vi "meas01.vi"() -> ()   [LabVIEW 2015]
uses:
  <vilib>/DAQmx/write.llb/DAQmx Write (Analog Wfm 1Chan NSamp).vi
  <vilib>/DAQmx/create/channels.llb/DAQmx Create Channel (AO-Voltage-Basic).vi
  <vilib>/DAQmx/configure/timing.llb/DAQmx Timing (Sample Clock).vi
  <vilib>/DAQmx/miscellaneous.llb/DAQmx Fill In Error Info.vi
  <vilib>/DAQmx/create/channels.llb/DAQmx Create Channel (CO-Pulse Generation-Frequency).vi
  <vilib>/DAQmx/configure/timing.llb/DAQmx Timing (Implicit).vi
  <vilib>/Utility/file.llb/Write Delimited Spreadsheet (DBL).vi
  <vilib>/measure/NI_MABase.lvlib
panel:
  in  "Vertical Coupling (1: DC)":i32(ring)=1 items=["AC", "DC", "Ground"]
  out "Waveform Data":waveform(dbl)(graph)
  out "Log-Log Frequency and Gain":cluster{"Y":dbl[], "Y":dbl[]}[](graph)
  out "freq in":dbl
  out "Loop #":i32
  out "detected amplitude":dbl format="%.2p"
  out "detected frequency":dbl format="%.2p"
  in  "Trigger Level (0.0 V)":dbl
  in  "Trigger Mode (0: Auto)":i32(ring) items=["Auto", "Normal"]
  in  "VISA resource name":refnum<visa-resource-name>
  in  "# Points":dbl
  in  "Highest Freq":dbl
  in  "Lowest Freq":dbl
  in  "Frequency (Hz)":dbl
  in  "Stop Clock":bool
  in  "Run":bool
  in  "stop":bool
  in  "physical channels":tag
  out "Amplitude":dbl
  in  "Amplitude":dbl(knob) scale=0.0..5.0
  in  "signal type":T1(ring)
  # "Clock"
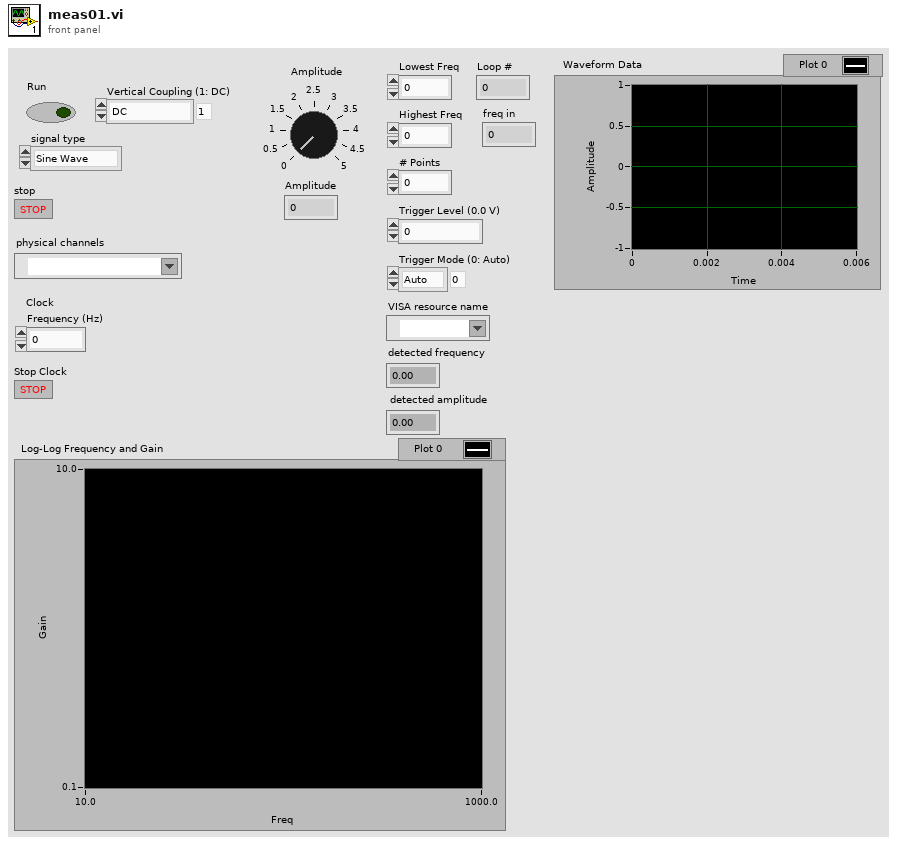
[diagram p1: front panel]
types:
  T1 = enum16{"Sine Wave", "Triangle Wave", "Square Wave", "Sawtooth Wave"}
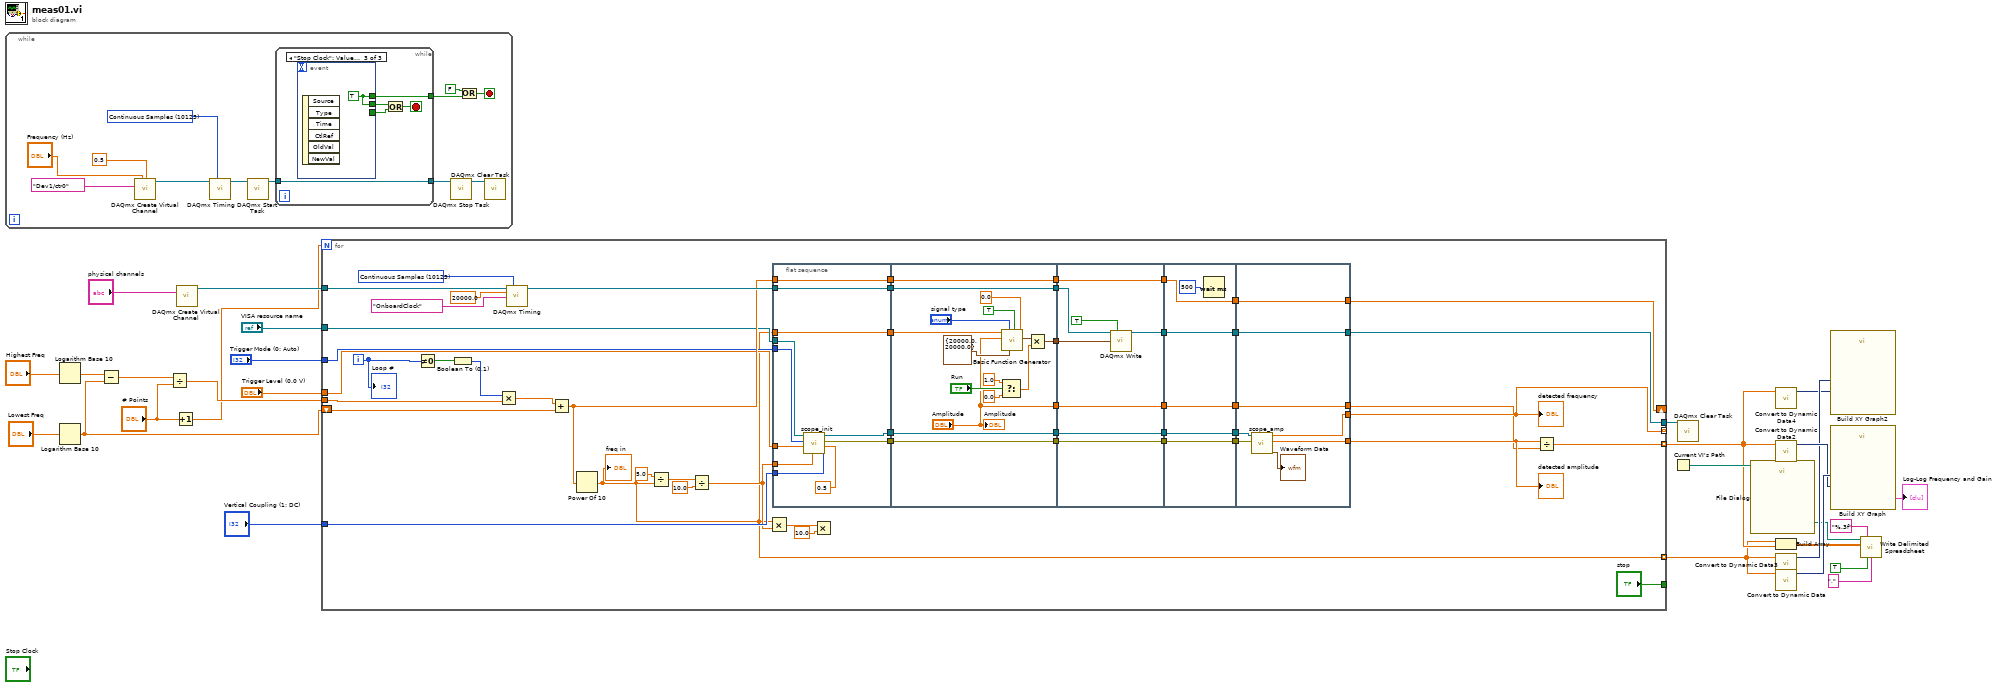
[diagram p0: block diagram]
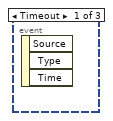
[diagram p2: hidden frame]
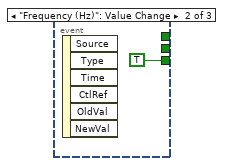
[diagram p3: hidden frame]
diagram:
  n1 = while {
    stop <- w32 stop-if-true
    w38 = 10123 items=["Finite Samples"=10178, "Continuous Samples"=10123, "Hardware Timed Single Point"=12522] ("sample mode")
    n2 = call-poly <vilib>:"DAQmx Create Virtual Channel.vi"("frequency"="Frequency (Hz)", "duty cycle"=0.5, "counter"=tag "Dev1/ctr0") -> ("task out"=w37:refnum<k21>)  [unwired: 11 in, 1 out]
    n3 = call-poly <vilib>:"DAQmx Timing.vi"("task/channels in"=w37, "sample mode"=w38) -> ("task out"=w36:refnum<k21>)  [unwired: 12 in, 1 out]
    n4 = call <vilib>:"DAQmx Start Task.vi"("task/channels in"=w36) -> ("task out"=w35:refnum<k21>)  [unwired: 13 in, 1 out]
    n5 = while {
      tunnel: w35 -> [w45]
      tunnel: [w45] -> w34
      tunnel: [w41] -> w31
      stop <- w42 stop-if-true
      n6 = event shown="[2] \"Stop Clock\": Value Change" {
        selector: _ -> [_ _ _]
        dyn-events: _ -> [_ _ _]
        timeout: _ -> [_ _ _]
        tunnel: [_ TRUE _] -> w43
        tunnel: [_ _ w47] -> w44
        tunnel: [_ _ w47] -> w41
        event Timeout {
          n7 = event-data() -> ()  [unwired: 1 in, 3 out]
        }
        event "Frequency (Hz)": Value Change {
          n8 = event-data() -> ()  [unwired: 1 in, 6 out]
        }
        event "Stop Clock": Value Change {
          w47 = TRUE
          n9 = event-data() -> ()  [unwired: 1 in, 6 out]
        }
      }
      n10 = Or(x=w44, y=w43) -> (x .or. y?=w42:bool)
    }
    n11 = call <vilib>:"DAQmx Stop Task.vi"("task/channels in"=w34) -> ("task out"=w33:refnum<k21>)  [unwired: 13 in, 1 out]
    n12 = Or(x=FALSE, y=w31) -> (x .or. y?=w32:bool)
    n13 = call <vilib>:"DAQmx Clear Task.vi"("task in"=w33) -> ()  [unwired: 14 in, 1 out]
  }
  n14 = Logarithm Base 10(1:"Highest Freq") -> (0:w20:dbl)
  n15 = Logarithm Base 10(1:"Lowest Freq") -> (0:w22:dbl)
  n16 = Subtract(x=w20, y=w22) -> (x-y=w24:dbl)
  n17 = Divide(x=w24, y="# Points") -> (x/y=w25:dbl)
  n18 = Increment(x="# Points") -> (x+1=w18:dbl)
  n19 = call-poly <vilib>:"DAQmx Create Virtual Channel.vi"("physical channels"="physical channels") -> ("task out"=w28:refnum<k21>)  [unwired: 13 in, 1 out]
  n20 = for {
    N: w18 -> [_]
    tunnel: w28 -> [w97]
    tunnel: [w74] -> w27
    tunnel: ["stop"] -> _
    tunnel: w25 -> [w92]
    tunnel: [w90] -> w2 mode=indexing
    tunnel: [w85] -> _ mode=indexing
    shift-right: [w66] -> _
    shift-left: w22 -> [w89]
    tunnel: "Trigger Level (0.0 V)" -> [w59]
    tunnel: "Trigger Mode (0: Auto)" -> [w61]
    tunnel: "VISA resource name" -> [w60]
    tunnel: "Vertical Coupling (1: DC)" -> [w58]
    tunnel: [w54] -> w1 mode=indexing
    i -> [w87]
    w94 = 10123 items=["Finite Samples"=10178, "Continuous Samples"=10123, "Hardware Timed Single Point"=12522] ("sample mode")
    n21 = Not Equal To 0?(x=w87) -> (x != 0?=w88:bool)
    n22 = Boolean To (0,1)(Boolean=w88) -> (0, 1=w86:i16)
    n23 = Multiply(x=w86, y=w92) -> (x*y=w91:dbl)
    n24 = call-poly <vilib>:"DAQmx Timing.vi"("task/channels in"=w97, "sample mode"=w94, "rate"=20000.0, "source"=tag "OnboardClock") -> ("task out"=w95:refnum<k21>)  [unwired: 10 in, 1 out]
    n25 = Add(x=w91, y=w89) -> (x+y=w67:dbl)
    n26 = Power Of 10(x=w67) -> (10^x=w54:dbl)
    "freq in" <- w54
    n27 = Divide(x=5.0, y=w54) -> (x/y=w78:dbl)
    n28 = Divide(x=w78, y=10.0) -> (x/y=w57:dbl)
    n29 = Multiply(x=w54, y=w57) -> (x*y=w56:dbl)
    n30 = flat-sequence {
      tunnel: w95 -> [w109]
      tunnel: [w109] -> w73
      tunnel: [w106] -> w72
      tunnel: [w105] -> w71
      tunnel: [w108] -> w68
      tunnel: w67 -> [w108]
      tunnel: [w107] -> w62
      tunnel: w54 -> [w107]
      tunnel: w61 -> [w101]
      tunnel: w60 -> [w104]
      tunnel: w59 -> [w102]
      tunnel: w57 -> [w103]
      tunnel: w58 -> [w99]
      tunnel: [w125] -> w53
      tunnel: [w124] -> w52
      tunnel: [w123] -> w51
      tunnel: w73 -> [w125]
      tunnel: w72 -> [w124]
      tunnel: w71 -> [w123]
      tunnel: [w122] -> w50
      tunnel: w68 -> [w122]
      tunnel: ["Amplitude"] -> w49
      tunnel: w62 -> [w121]
      tunnel: [w110] -> w48
      tunnel: [w132] -> w83
      tunnel: [w131] -> w81
      tunnel: [w130] -> w75
      tunnel: w53 -> [w133]
      tunnel: w52 -> [w132]
      tunnel: w51 -> [w131]
      tunnel: [w129] -> w69
      tunnel: w50 -> [w129]
      tunnel: [w128] -> w64
      tunnel: w49 -> [w128]
      tunnel: w48 -> [w126]
      tunnel: w83 -> [w139]
      tunnel: [w139] -> w82
      tunnel: w81 -> [w138]
      tunnel: [w138] -> w80
      tunnel: [w136] -> w76
      tunnel: w75 -> [w136]
      tunnel: [w135] -> w70
      tunnel: w69 -> [w135]
      tunnel: [w134] -> w65
      tunnel: w64 -> [w134]
      tunnel: w82 -> [w147]
      tunnel: w80 -> [w146]
      tunnel: [w145] -> w85
      tunnel: [w144] -> w84
      tunnel: [w143] -> w74
      tunnel: w76 -> [w143]
      tunnel: [w142] -> w66
      tunnel: w70 -> [w142]
      tunnel: [w141] -> w63
      tunnel: w65 -> [w141]
      frame #0 {
        n31 = call "scope_init.vi"("Vertical Coupling (1: DC)"=w99, "Vertical Range (10.0 V/div)"=0.5, "Timebase (0.0005 s)"=w103, "Trigger Level (0.0 V)"=w102, "Trigger Mode (0: Auto)"=w101, "VISA resource name"=w104) -> ("error out"=w105:errorcluster, "VISA resource name out"=w106:refnum<visa-resource-name>)  [unwired: 4 in]
      }
      frame #1 {
        n32 = Select(t=1.0, s="Run", f=0.0) -> (s? t:f=w116:dbl)
        n33 = call <vilib>:"Basic Function Generator.vi"("offset"=0.0, "reset signal"=TRUE, "sampling info"=cluster{"Fs":dbl, "#s":dbl} {"Fs"=20000.0, "#s"=20000.0}, "signal type"="signal type", "amplitude"="Amplitude", "frequency"=w121) -> ("signal out"=w120:waveform(dbl))  [unwired: 3 in, 2 out]
        n34 = Multiply(x=w120, y=w116) -> (x*y=w110:waveform(dbl))
        "Amplitude" <- "Amplitude"
      }
      frame #2 {
        n35 = call-poly <vilib>:"DAQmx Write.vi"("task/channels in"=w133, "auto start"=TRUE, "data"=w126) -> ("task out"=w130:refnum<k21>)  [unwired: 10 in, 2 out]
      }
      frame #3 {
        n36 = Wait (ms)(milliseconds to wait=u32 500) -> ()  [unwired: 1 out]
      }
      frame #4 {
        n37 = call "scope_amp.vi"("error in (no error)"=w146, "VISA resource name"=w147) -> ("Waveform Data"=→"Waveform Data":waveform(dbl), "detected amplitude"=w144:dbl, "detected frequency"=w145:dbl)  [unwired: 6 in, 1 out]
      }
    }
    n38 = Multiply(x=w56, y=10.0) -> ()  [unwired: 1 out]
    n39 = Divide(x=w84, y=w63) -> (x/y=w90:dbl)
    "detected frequency" <- w85
    "detected amplitude" <- w84
    "Loop #" <- w87
  }
  n40 = Current VI's Path() -> (path=w9:path)
  n41 = call <vilib>:"DAQmx Clear Task.vi"("task in"=w27) -> ()  [unwired: 14 in, 1 out]
  n42 = call "File Dialog"("start path"=w9) -> ("selected path"=w7:path)  [unwired: 11 in, 3 out]
  n43 = call "Convert to Dynamic Data4"("Array"=w2) -> ("Dynamic Data Type"=w13:dynamicdata)  [unwired: 3 in]
  n44 = call "Convert to Dynamic Data2"("Array"=w2) -> ("Dynamic Data Type"=w15:dynamicdata)  [unwired: 3 in]
  n45 = Build Array(w1, w2) -> (w4:dbl[][])
  n46 = call "Convert to Dynamic Data3"("Array"=w1) -> ("Dynamic Data Type"=w14:dynamicdata)  [unwired: 3 in]
  n47 = call "Convert to Dynamic Data"("Array"=w1) -> ("Dynamic Data Type"=w16:dynamicdata)  [unwired: 3 in]
  n48 = call "Build XY Graph2"("Y Input"=w13, "X Input"=w14) -> ()  [unwired: 8 in, 2 out]
  n49 = call "Build XY Graph"("Y Input"=w15, "X Input"=w16) -> ("XY Graph"=→"Log-Log Frequency and Gain":cluster{"X":dbl[], "Y":dbl[]}[])  [unwired: 8 in, 1 out]
  n50 = call-poly <vilib>:"Write Delimited Spreadsheet.vi"("file path (dialog if empty)"=w7, "format (%.3f)"="%.3f", "2D data"=w4, "transpose? (F)"=TRUE ("transpose? (no:F)"), "delimiter (\\t)"="," ("delimiter (\\t)")) -> ()  [unwired: 9 in, 2 out]
